vi "Profile Creation.vi"() -> ()   [LabVIEW 2018]
uses:
  Controls/Profile Create Cluster.ctl
panel:
  in  "Select Profile":path
  in  "Profile Creation":T1[](array[typedef])
  out "Headline":string
  in  "Save Button":bool
  # "Auto Cycle Profile Creation"
  # "Start RPM"
  # "End RPM"
  # "Ramp Time"
  # "Torque Value"
  # "Operation"
  # "Stable Time"
  # "Datalog"
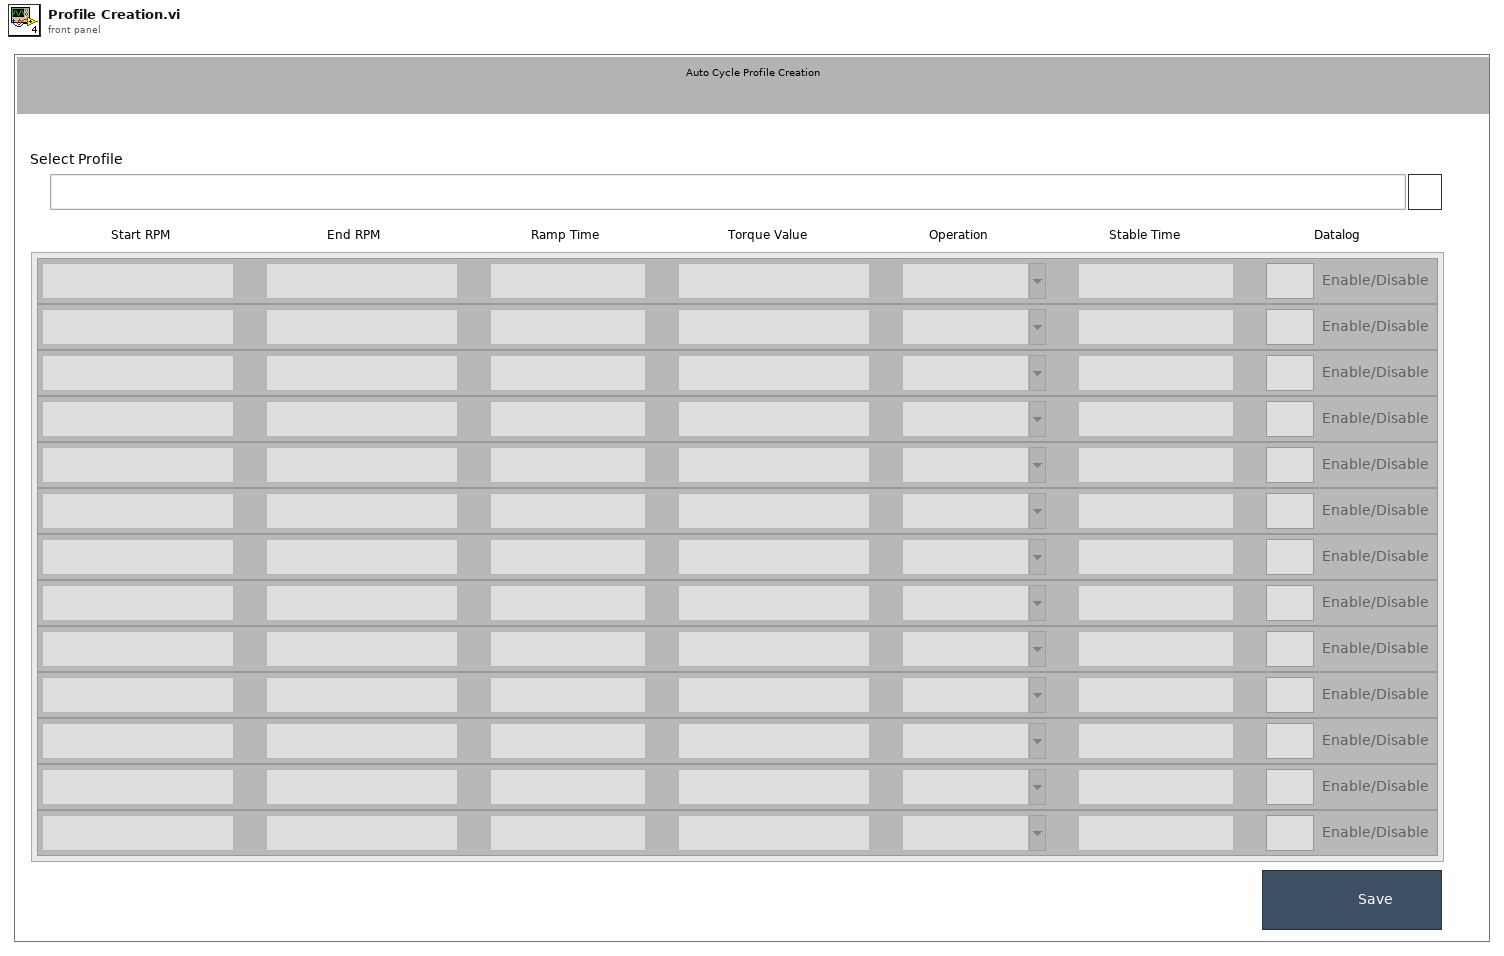
[diagram p1: front panel]
types:
  T1 = typedef "Profile Create Cluster.ctl" = cluster{"Start RPM":string, "End RPM":string, "Operation":string, "Torque Value":string, "Datalog":bool, "Ramp Time":string, "Stable Time":string}
  T2 = enum32{"Invalid", "Standard", "Closed", "Hidden", "Minimized", "Maximized"}
  T3 = enum32{"invalid app kind", "Development System", "Run Time System", "Student Edition", "Embedded LabVIEW", "Evaluation", "Custom"}
  T4 = cluster{"Core":cluster{"Current VI Reference":refnum<vi>, "Close Panel on Exit?":bool}, "Your Boolean data":bool, "Your string data":string, "Profile Creation":T1[], "File paths":cluster{"Base file path":path, "Model File path":path}, "Select Profile":path}
  T5 = cluster{"Base file path":path, "Model File path":path}
  T6 = cluster{"Current VI Reference":refnum<vi>, "Close Panel on Exit?":bool}
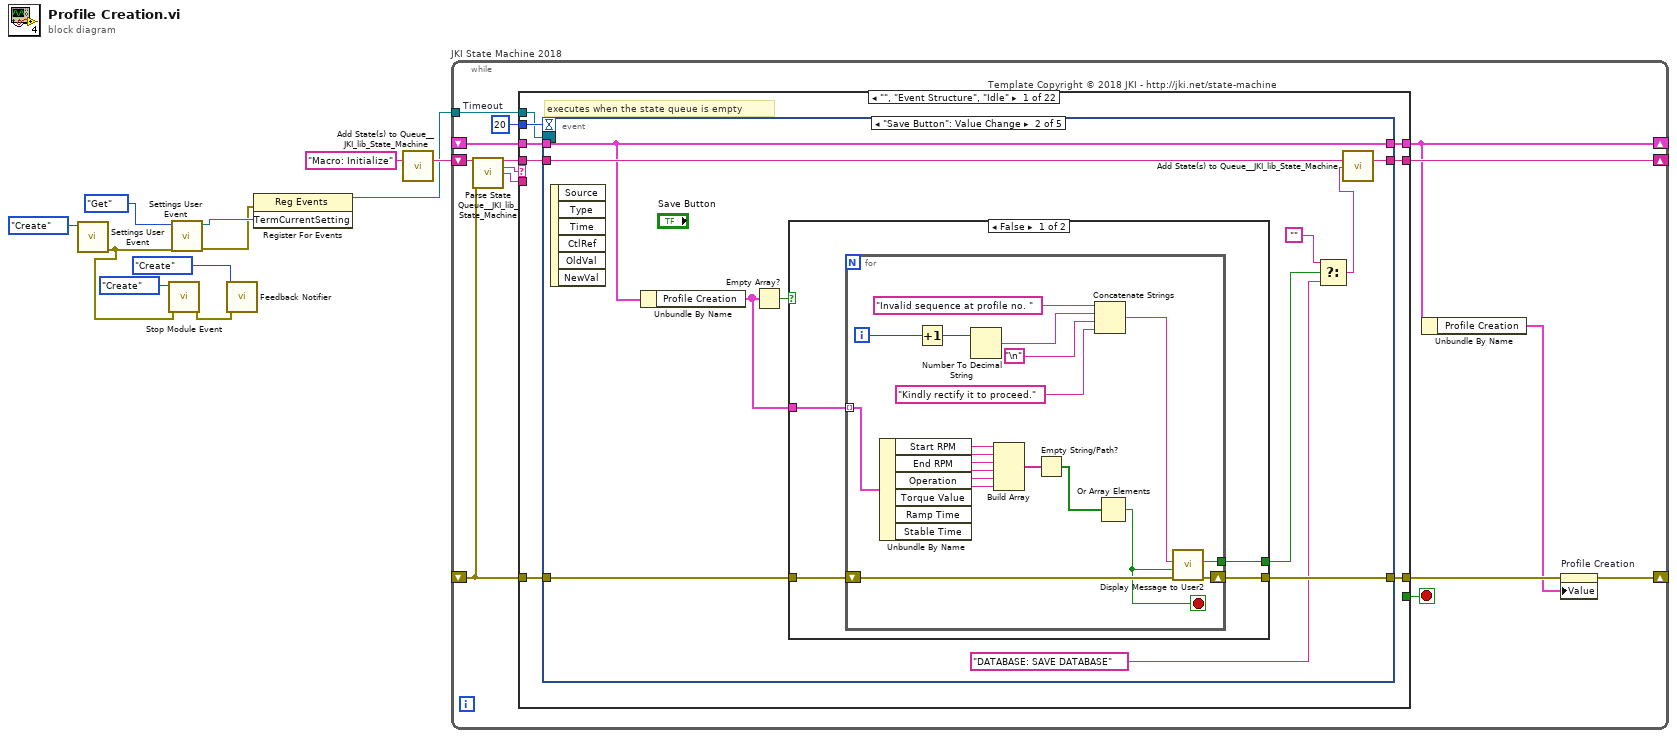
[diagram p0: block diagram]
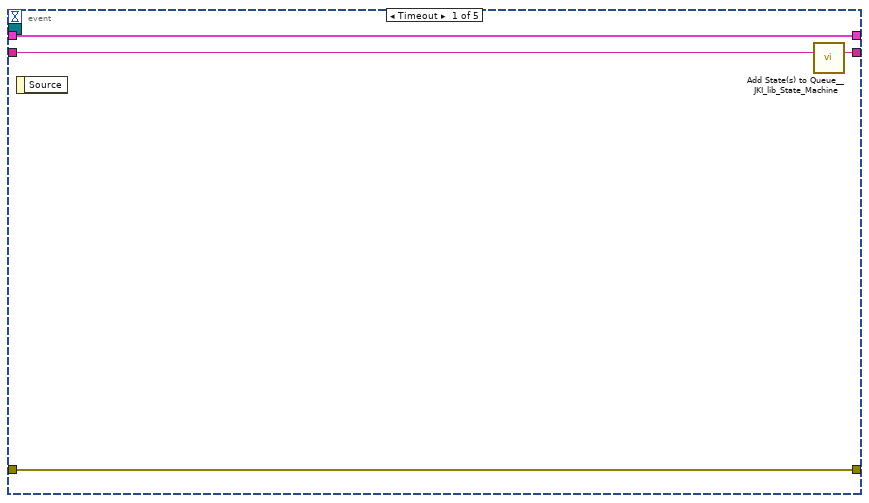
[diagram p2: hidden frame]
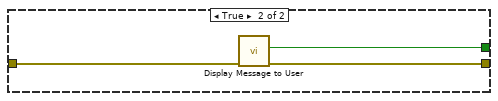
[diagram p3: hidden frame]
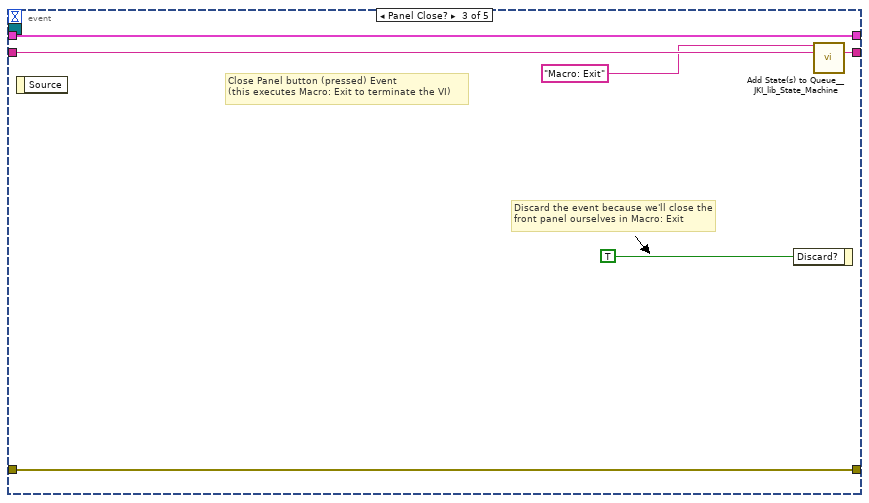
[diagram p4: hidden frame]
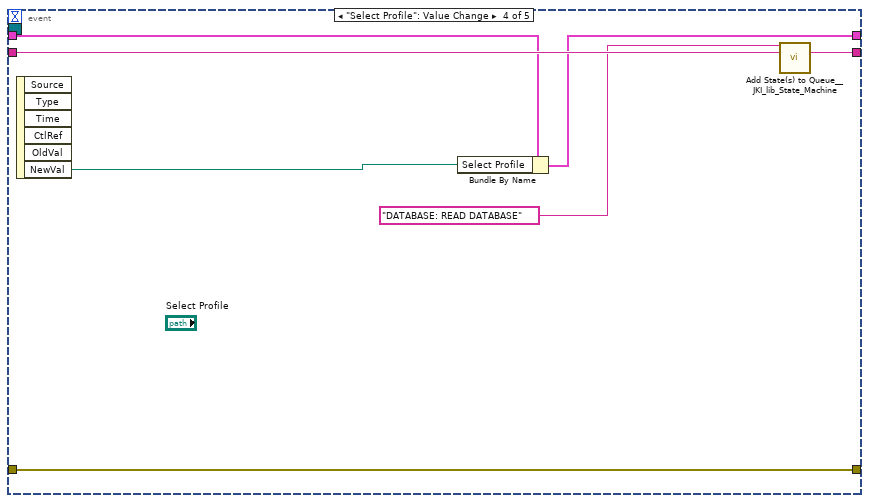
[diagram p5: hidden frame]
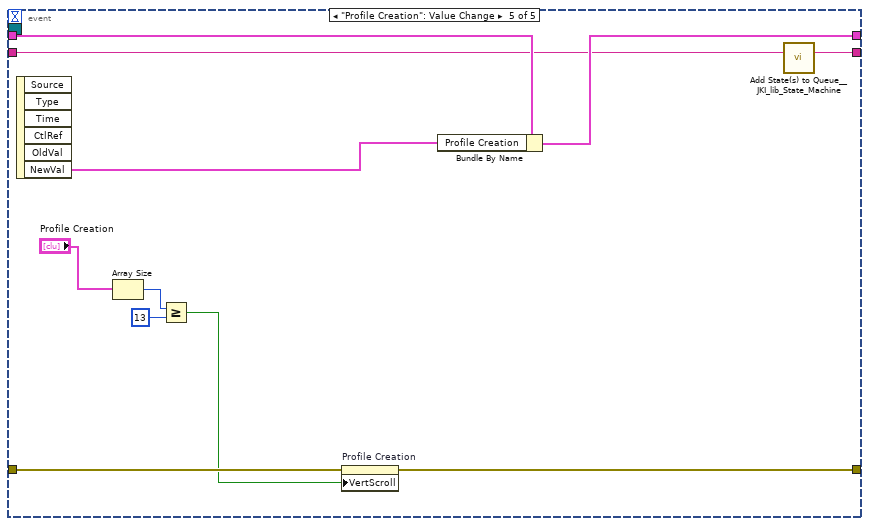
[diagram p6: hidden frame]
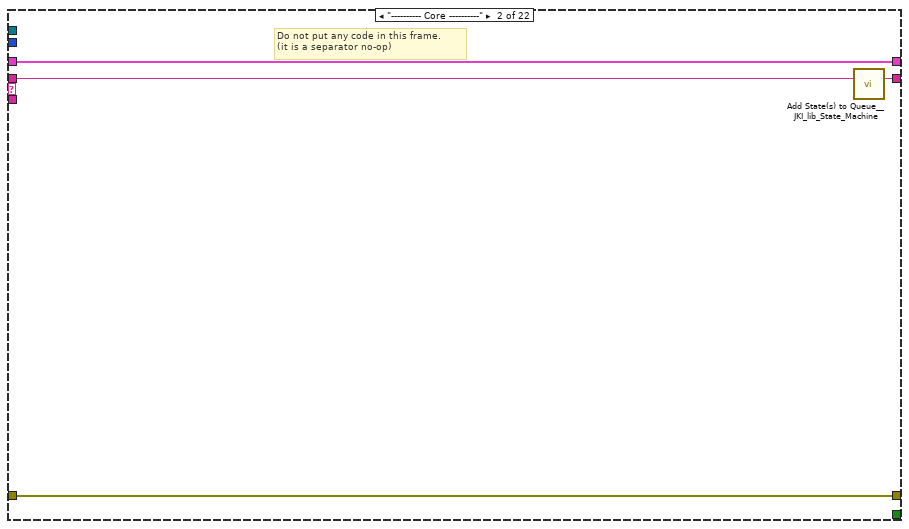
[diagram p7: hidden frame]
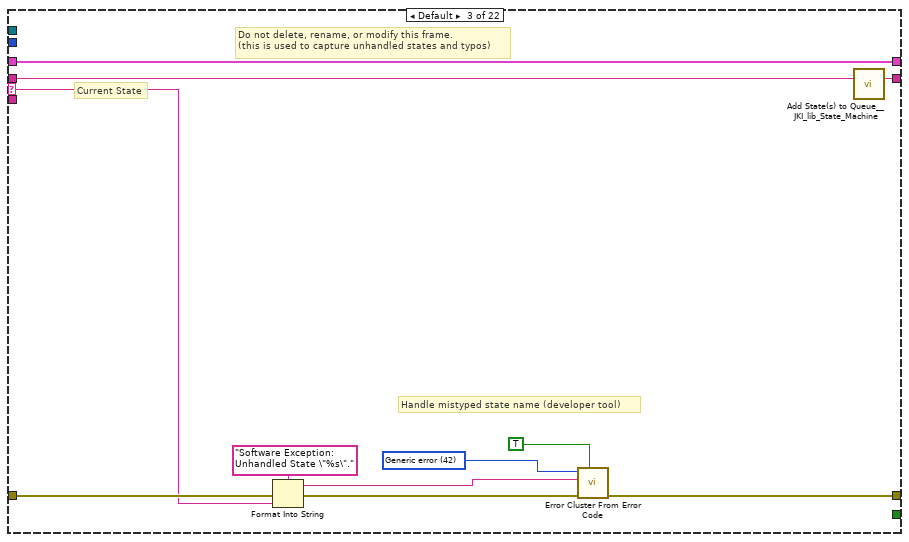
[diagram p8: hidden frame]
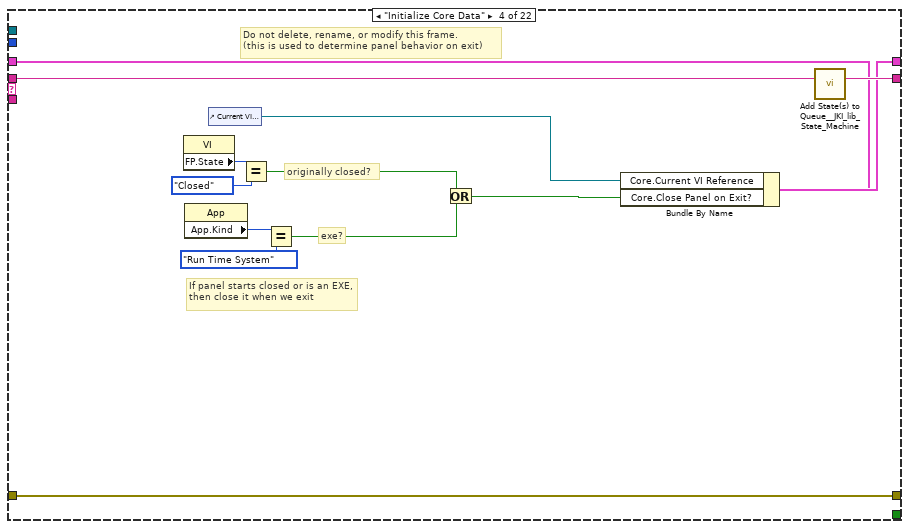
[diagram p9: hidden frame]
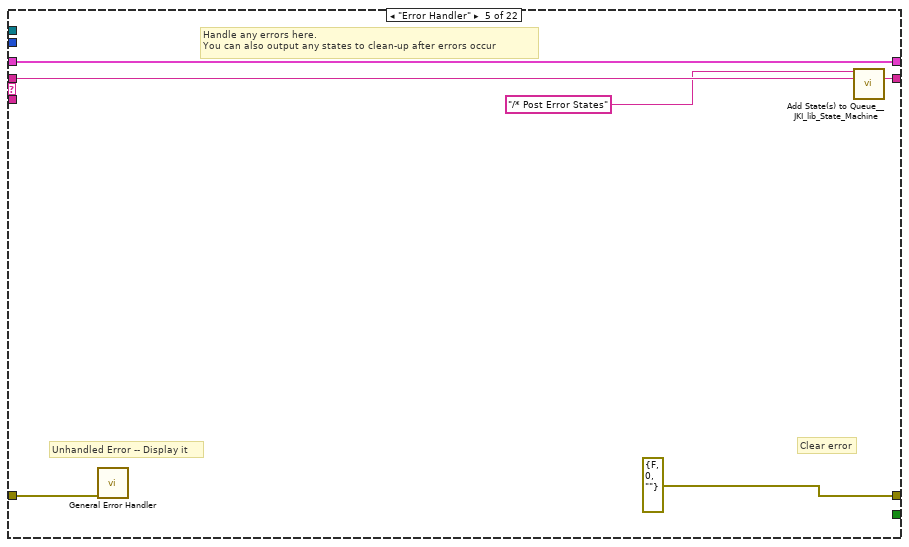
[diagram p10: hidden frame]
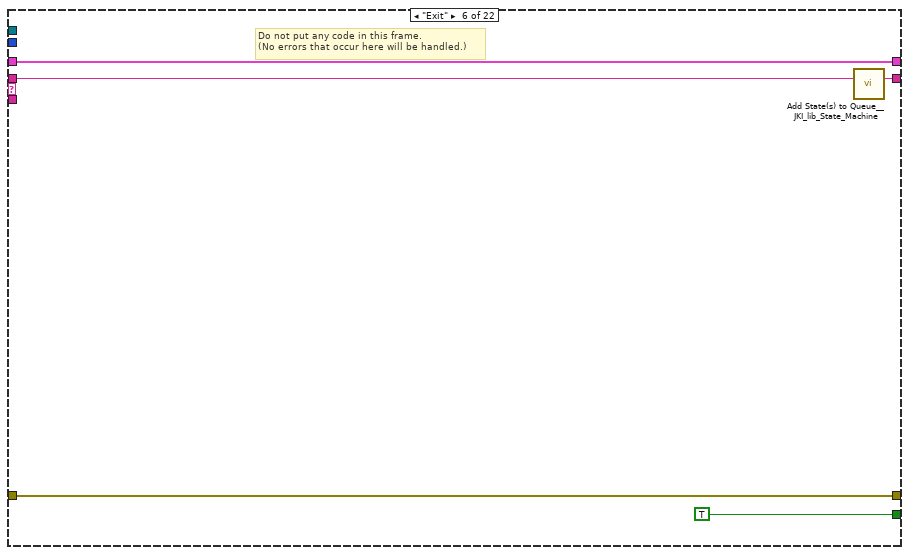
[diagram p11: hidden frame]
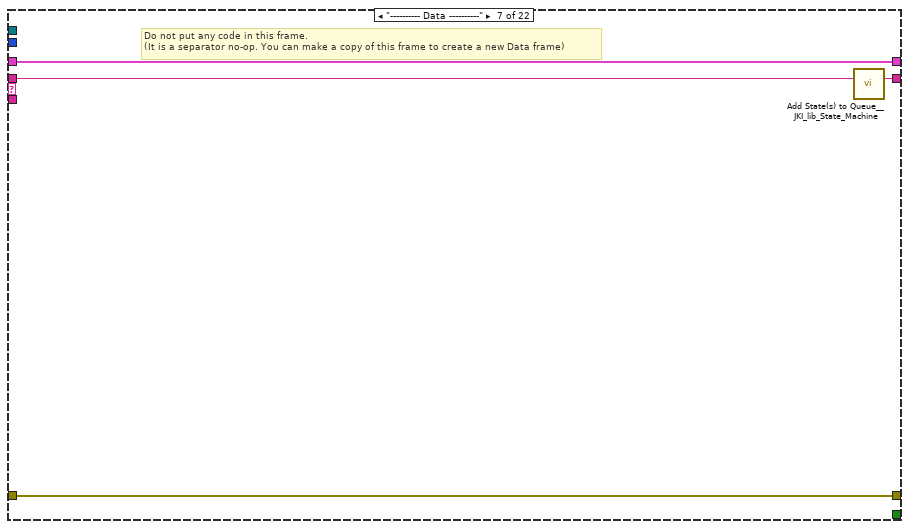
[diagram p12: hidden frame]
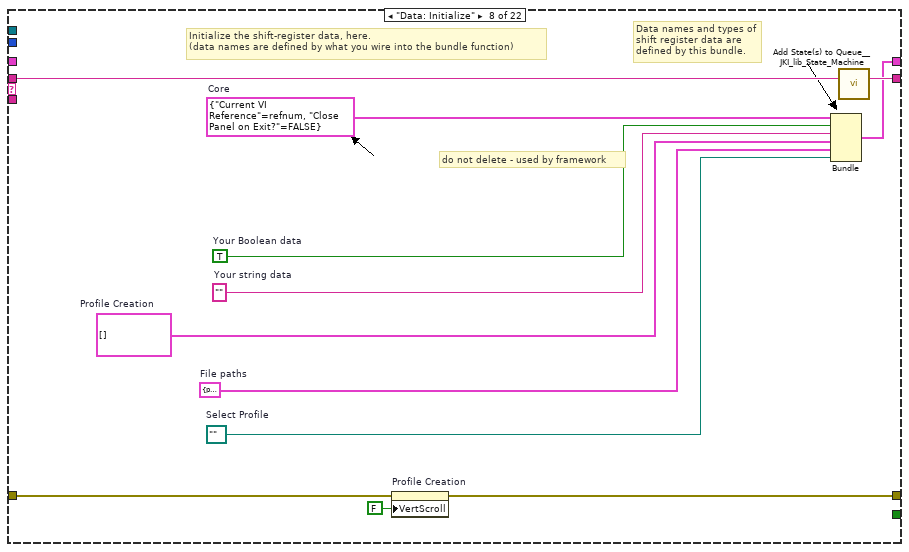
[diagram p13: hidden frame]
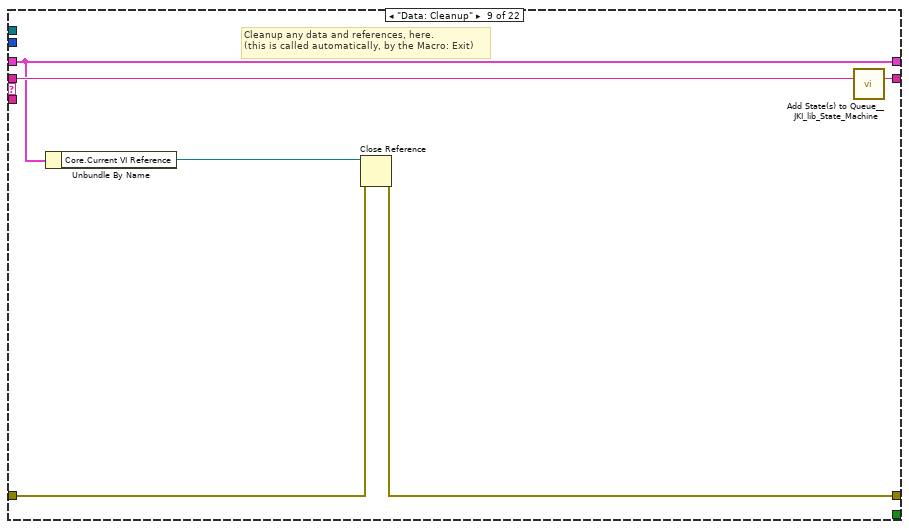
[diagram p14: hidden frame]
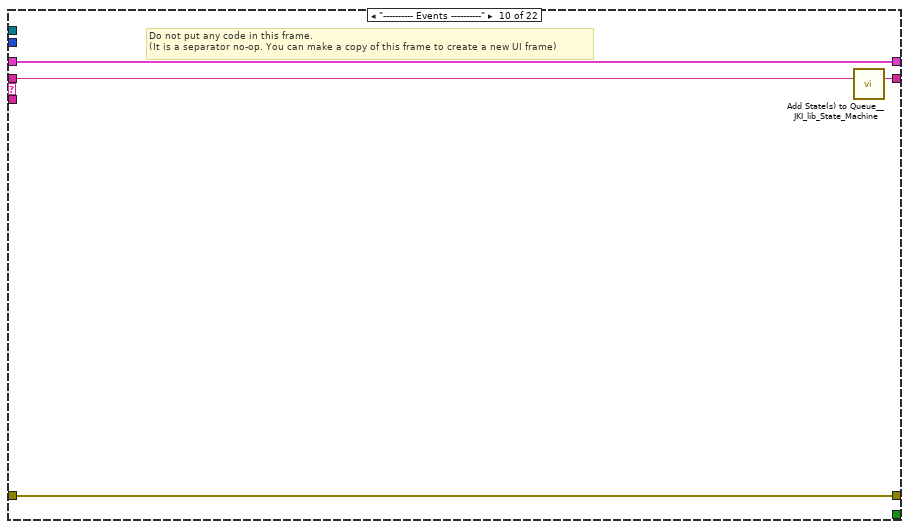
[diagram p15: hidden frame]
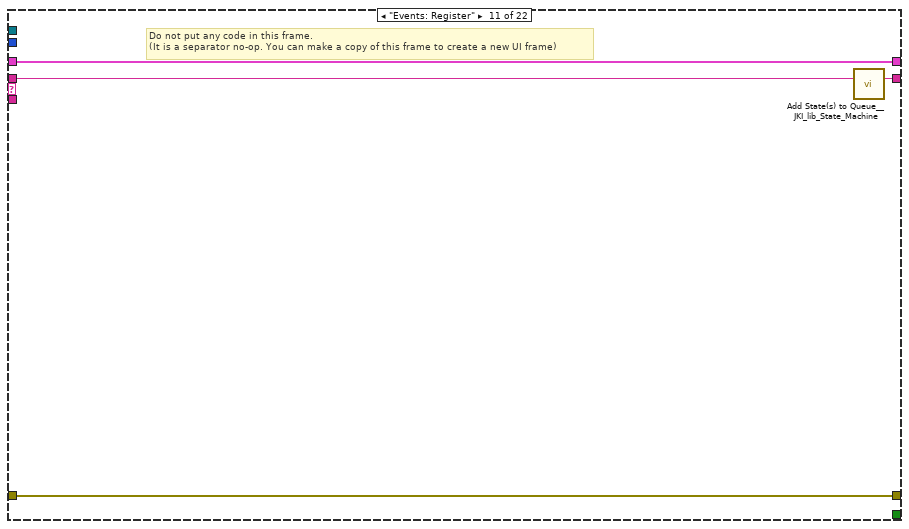
[diagram p16: hidden frame]
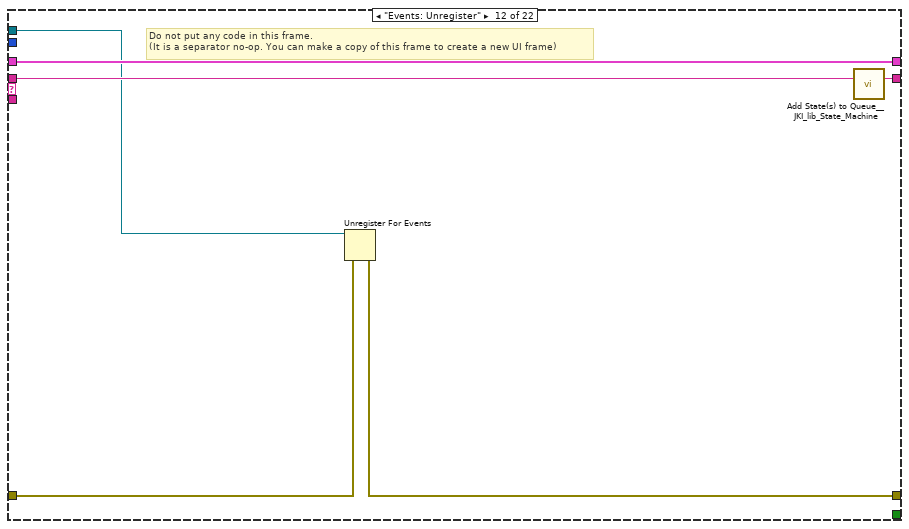
[diagram p17: hidden frame]
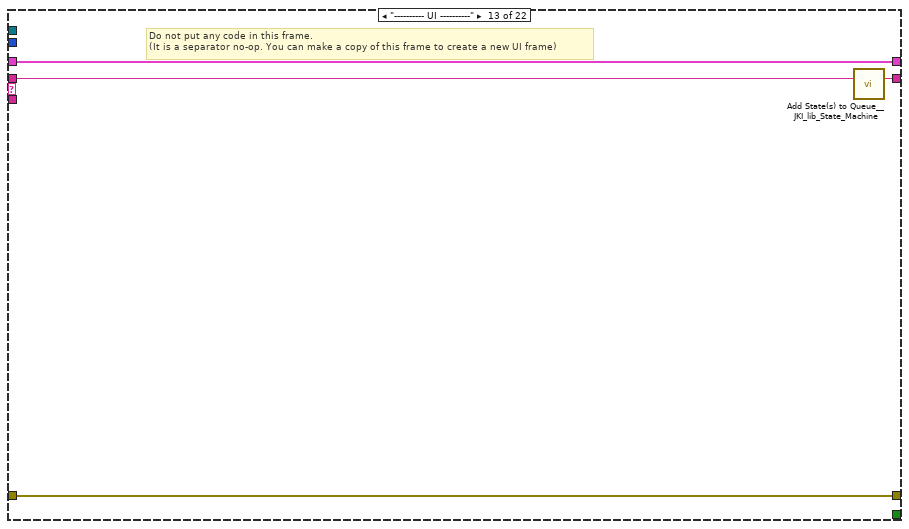
[diagram p18: hidden frame]
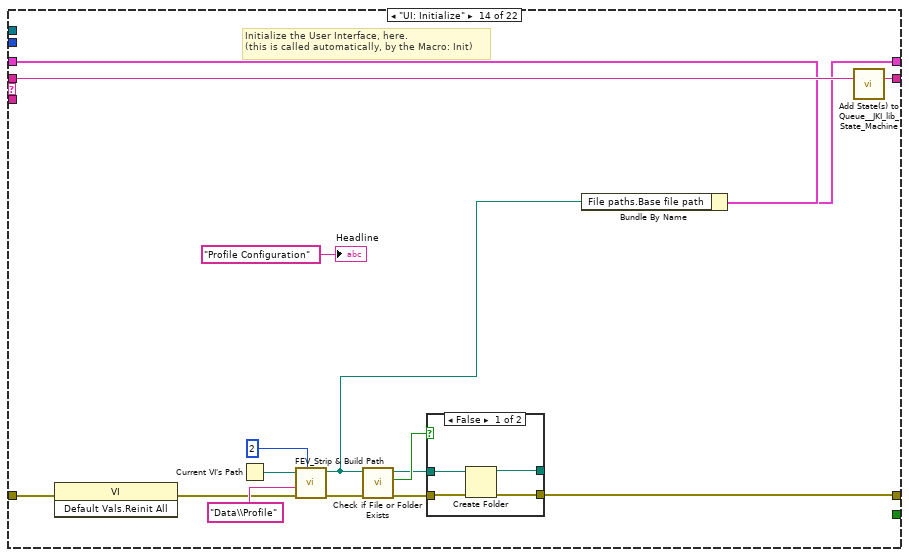
[diagram p19: hidden frame]
diagram:
  n1 = call "Settings User Event.vi"("Action"=enum16{"Create", "Get", "Destroy"}."Create") -> ("error out"=w4:errorcluster)  [unwired: 9 in, 1 out]
  n2 = call "Stop Module Event.vi"("error in (no error)"=w4, "Action"=enum16{"Create", "Get", "Destroy"}."Create") -> ("error out"=w3:errorcluster)  [unwired: 8 in, 1 out]
  n3 = call "Settings User Event.vi"("error in (no error)"=w4, "Action"=enum16{"Create", "Get", "Destroy"}."Get") -> ("error out"=w6:errorcluster, "TermCurrentSetting"=w7:refnum<user-event>)  [unwired: 8 in]
  n4 = call "Feedback Notifier.vi"("error in (no error)"=w3, "Action"=enum16{"Create", "Get", "Destroy"}."Create") -> ()  [unwired: 8 in, 2 out]
  n5 = register-events(error in=w6, w7) -> (reference out=w1:refnum<event-registration>)  [unwired: 1 in, 1 out]
  n6 = call <vilib>:"Add State(s) to Queue__JKI_lib_State_Machine.vi"("State(s) in (\"\")"="Macro: Initialize") -> ("States Out"=w11:string)  [unwired: 14 in]
  n7 = while "JKI State Machine 2018" {
    shift-right: [w13] -> _
    shift-left: _ -> [w19]
    shift-right: [w14] -> _
    shift-left: _ -> [w17]
    shift-right: [w21] -> _
    shift-left: w11 -> [w22]
    tunnel: w1 -> [w16]
    stop <- w20 stop-if-true
    w18 = 20  # Timeout
    # "Template Copyright © 2018 JKI - http://jki.net/state-machine"
    n8 = call <vilib>:"Parse State Queue__JKI_lib_State_Machine.vi"("State Queue"=w22, "Error In (no error)"=w17) -> ("Remaining States"=w24:string, "Current State"=w25:string, "Arguments"=w23:string)  [unwired: 11 in]
    n9 = case shown="\"\", \"Event Structure\", \"Idle\"" w25 {
      selector: w25 -> [_ _ w104 _ _ _ _ _ _ _ _ _ _ _ _ _ _ _ _ _ _ _]
      tunnel: w24 -> [w33 w103 w108 w127 w133 w138 w142 w154 w160 w164 w168 w174 w178 w194 w206 w217 w286 w291 w301 w305 w316 w340]
      tunnel: w23 -> [_ _ _ _ _ _ _ _ _ _ _ _ _ _ w201 w211 _ _ _ _ _ _]
      tunnel: w19 -> [w31 w100 w106 w120 w130 w136 w139 _ w155 w161 w166 w172 w175 w189 w204 w213 w283 w288 w298 w302 w314 w338]
      tunnel: [w30 w101 w110 w124 errorcluster {"status"=FALSE, "code"=0, "source"=""} ("error out") w135 w140 w143 w156 w162 w165 w169 w176 w179 w202 w214 w284 w289 w299 w303 w313 w331] -> w15
      tunnel: w17 -> [w29 w101 w109 w124 w129 w135 w140 w144 w157 w162 w165 w170 w176 w187 w203 w215 w284 w289 w299 w303 w310 w336]
      tunnel: [w32 w102 w107 w126 w132 w137 w141 w153 w159 w163 w167 w173 w177 w193 w205 w216 w285 w290 w300 w304 w315 w339] -> w21
      tunnel: [_ _ _ _ _ TRUE _ _ _ _ _ _ _ _ _ _ _ _ _ _ _ _] -> w20
      tunnel: [w28 w100 w106 w125 w130 w136 w139 w152 w155 w161 w166 w172 w175 w188 w204 w213 w283 w288 w298 w302 w314 w337] -> w13
      tunnel: w18 -> [w27 _ _ _ _ _ _ _ _ _ _ _ _ _ _ _ _ _ _ _ _ _]
      tunnel: w16 -> [w26 _ _ _ _ _ _ _ _ _ _ w171 _ _ _ _ _ _ _ _ _ _]
      frame "", "Event Structure", "Idle" {
        # "executes when the state queue is empty"
        n10 = event shown="[1] \"Save Button\": Value Change" {
          selector: w26 -> [_ _ _ _ _]
          dyn-events: _ -> [_ _ _ _ _]
          timeout: w27 -> [_ _ _ _ _]
          tunnel: w33 -> [w37 w47 w81 w86 w96]
          tunnel: [w36 w48 w80 w87 w97] -> w32
          tunnel: w31 -> [w34 w46 w78 w85 w99]
          tunnel: [w35 w43 w79 w88 w91] -> w30
          tunnel: w29 -> [w35 w45 w79 w88 w92]
          tunnel: [w34 w46 w78 w84 w98] -> w28
          event Timeout {
            n11 = event-data() -> ()  [unwired: 1 in, 1 out]
            n12 = call <vilib>:"Add State(s) to Queue__JKI_lib_State_Machine.vi"("State(s) in (\"\")"=w37) -> ("States Out"=w36:string)  [unwired: 14 in]
          }
          event "Save Button": Value Change {
            n13 = event-data() -> ()  [unwired: 1 in, 6 out]
            n14 = Unbundle By Name(w46) -> ("Profile Creation"=w42:T1[])
            n15 = Empty Array?(array=w42) -> (empty?=w44:bool)
            n16 = case shown="False" w44 {
              tunnel: w45 -> [w51 w75]
              tunnel: [w50 w74] -> w43
              tunnel: w42 -> [w52 _]
              tunnel: [w49 w73] -> w41
              frame False {
                n17 = for {
                  tunnel: w52 -> [w72] mode=indexing
                  shift-right: [w63] -> w50
                  shift-left: w51 -> [w64]
                  tunnel: [w53] -> w49
                  i -> [w60]
                  stop <- w61 stop-if-true
                  n18 = Unbundle By Name(w72) -> ("Start RPM"=w71:string, "End RPM"=w70:string, "Operation"=w69:string, "Torque Value"=w68:string, "Ramp Time"=w67:string, "Stable Time"=w66:string)
                  n19 = Increment(x=w60) -> (x+1=w59:i32)
                  n20 = Number To Decimal String(number=w59) -> (decimal integer string=w58:string)  [unwired: 1 in]
                  n21 = Build Array(w71, w70, w69, w68, w67, w66) -> (w65:string[])
                  n22 = Empty String/Path?(string/path=w65) -> (empty?=w62:bool[])
                  n23 = Concatenate Strings("Invalid sequence at profile no. " ("string"), w58, "\n", "Kindly rectify it to proceed." ("string")) -> (w55:string)
                  n24 = Or Array Elements(Boolean array=w62) -> (logical OR=w61:bool)
                  n25 = call "Display Message to User2"("error in (no error)"=w64, "Enable"=w61, "Message"=w55) -> ("error out"=w63:errorcluster, "OK"=w53:bool)  [unwired: 7 in]
                }
              }
              frame True {
                n26 = call "Display Message to User"("error in (no error)"=w75) -> ("error out"=w74:errorcluster, "OK"=w73:bool)  [unwired: 9 in]
              }
            }
            n27 = Select(t="", s=w41, f="DATABASE: SAVE DATABASE") -> (s? t:f=w38:string)
            n28 = call <vilib>:"Add State(s) to Queue__JKI_lib_State_Machine.vi"("State(s) in (\"\")"=w47, "State(s) at Back (\"\")"=w38) -> ("States Out"=w48:string)  [unwired: 13 in]
          }
          event Panel Close? {
            # "Discard the event because we'll close the front panel ourselves in Macro: Exit"
            # "Close Panel button (pressed) Event\n(this executes Macro: Exit to terminate the VI)"
            n29 = event-data() -> ()  [unwired: 1 in, 1 out]
            n30 = event-data("Discard?"=TRUE) -> ()  [unwired: 1 in, 1 out]
            n31 = call <vilib>:"Add State(s) to Queue__JKI_lib_State_Machine.vi"("State(s) in Front (\"\")"="Macro: Exit", "State(s) in (\"\")"=w81) -> ("States Out"=w80:string)  [unwired: 13 in]
          }
          event "Select Profile": Value Change {
            n32 = event-data() -> ("NewVal"=w83:path)  [unwired: 1 in, 5 out]
            n33 = Bundle By Name(cluster=w85, "Select Profile"=w83) -> (w84:T4)
            n34 = call <vilib>:"Add State(s) to Queue__JKI_lib_State_Machine.vi"("State(s) in Front (\"\")"="DATABASE: READ DATABASE" ("State(s) in Front (\"\")"), "State(s) in (\"\")"=w86) -> ("States Out"=w87:string)  [unwired: 13 in]
          }
          event "Profile Creation": Value Change {
            n35 = event-data() -> ("NewVal"=w89:T1[])  [unwired: 1 in, 5 out]
            n36 = Array Size(array="Profile Creation") -> (size(s)=w94:i32)
            n37 = Greater Or Equal?(x=w94, y=13) -> (x >= y?=w90:bool)
            n38 = property on="Profile Creation" class="Arr (strict)"(error in=w92, "VertScroll"=w90) -> (error out=w91:errorcluster)  [unwired: 1 in, 1 out]
            n39 = Bundle By Name(cluster=w99, "Profile Creation"=w89) -> (w98:T4)
            n40 = call <vilib>:"Add State(s) to Queue__JKI_lib_State_Machine.vi"("State(s) in (\"\")"=w96) -> ("States Out"=w97:string)  [unwired: 14 in]
          }
        }
      }
      frame "---------- Core ----------" {
        # "Do not put any code in this frame.\n(it is a separator no-op)"
        n41 = call <vilib>:"Add State(s) to Queue__JKI_lib_State_Machine.vi"("State(s) in (\"\")"=w103) -> ("States Out"=w102:string)  [unwired: 14 in]
      }
      frame Default {
        w113 = 42 items=["No error", "Argument error", "Memory is full", "Out of zone", "End of file", "File already open", "Generic file I/O error", "File not found", "File permission error", "Disk is full", "Duplicate path", "Too many files open", "System feature not enabled", "Resource file not found", "Cannot add resource", "Resource not found", "Image not found", "Image memory error", "Pen does not exist", "Config type invalid", "Config token not found", "Config parse error", "Config memory error", "Bad external code format", "Bad external code offset", "External code not present", "Null window", "Destroy window error", "Null menu", "Print aborted", "Bad print record", "Print driver error", "Windows error during printing", "Memory error during printing", "Print dialog error", "Generic print error", "Invalid device refnum", "Device not found", "Device parameter error", "Device unit error", "Cannot open device", "Device call aborted", "Generic error", "Cancelled by user", "Object ID too low", "Object ID too high", "Object not in heap", "Unknown heap", "Unknown object (invalid DefProc)", "Unknown object (DefProc not in table)", "Message out of range", "Invalid (null) method", "Unknown message", "Manager call not supported", "Bad address", "Network operation in progress", "Network operation timed out", "Connection is busy", "Network attribute not supported", "Network error", "Address in use", "System out of memory", "Connection aborted", "Connection refused", "Not connected", "Already connected", "Connection closed", "Initialization error (interapplication manager)", "Bad occurrence", "Wait on unbound occurrence handler", "Occurrence queue overflow", "Datalog type conflict", "Unused", "Unrecognized type (interapplication manager)", "Memory corrupt", "Failed to make temporary DLL", "Old CIN version", "Drag socket not found", "Failed to load drop-object", "Failed to register OLE object", "Failed to release OLE object", "Format specifier type mismatch", "Unknown format specifier", "Too few format specifiers", "Too many format specifiers", "Scan failed", "Newer CIN version", "Error converting to variant", "Runtime menu error", "Password tampered", "Variant attribute not found", "Incompatible variant data type", "Event data is not available", "Event Store is not present", "Occurrence is not found", "Event Queue is not created", "Event info is not available", "Refnum passed is NULL", "Error retrieving Class GUID", "Error retrieving CoClass GUID", "Error retrieving TypeLib GUID.", "Bad built application magic bytes.", "Specific driver is different from the specific driver associated with the Logical Name.", "There is no session opened to the class driver.", "Max Error", "MAX - Error with config objects", "MAX - Error loading configuration", "MAX - Group not supported"]
        # "Current State"
        # "Do not delete, rename, or modify this frame.\n(this is used to capture unhandled states and typos)"
        # "Handle mistyped state name (developer tool)"
        n42 = Format Into String(format string="Software Exception: Unhandled State \"%s\"." ("message"), error in=w109, w104) -> (resulting string=w112:string, error out=w111:errorcluster)  [unwired: 1 in]
        n43 = call <vilib>:"Error Cluster From Error Code.vi"("show call chain? (False)"=TRUE, "error in (no error)"=w111, "error message (\"\")"=w112, "error code (0)"=w113) -> ("error out"=w110:errorcluster)  [unwired: 5 in]
        n44 = call <vilib>:"Add State(s) to Queue__JKI_lib_State_Machine.vi"("State(s) in (\"\")"=w108) -> ("States Out"=w107:string)  [unwired: 14 in]
      }
      frame "Initialize Core Data" {
        # "Do not delete, rename, or modify this frame.\n(this is used to determine panel behavior on exit)"
        # "originally closed?"
        # "exe?"
        # "If panel starts closed or is an EXE, then close it when we exit"
        n45 = property class="VI"() -> ("FP.State"=w117:T2)  [unwired: 2 in, 2 out]
        n46 = property class="App"() -> ("App.Kind"=w123:T3)  [unwired: 2 in, 2 out]
        n47 = control-ref of="Current VI Reference"() -> (w118:refnum<vi>)
        n48 = Equal?(x=w117, y=T2."Closed" ("Front Panel Window:State")) -> (x = y?=w115:bool)
        n49 = Equal?(x=w123, y=T3."Run Time System" ("Application:Kind")) -> (x = y?=w121:bool)
        n50 = Or(x=w115, y=w121) -> (x .or. y?=w119:bool)
        n51 = Bundle By Name(cluster=w120, "Core.Current VI Reference"=w118, "Core.Close Panel on Exit?"=w119) -> (w125:T4)
        n52 = call <vilib>:"Add State(s) to Queue__JKI_lib_State_Machine.vi"("State(s) in (\"\")"=w127) -> ("States Out"=w126:string)  [unwired: 14 in]
      }
      frame "Error Handler" {
        # "Unhandled Error -- Display it"
        # "Handle any errors here.\nYou can also output any states to clean-up after errors occur"
        # "Clear error"
        n53 = call <vilib>:"General Error Handler.vi"("error in (no error)"=w129) -> ()  [unwired: 10 in, 5 out]
        n54 = call <vilib>:"Add State(s) to Queue__JKI_lib_State_Machine.vi"("State(s) in Front (\"\")"="/* Post Error States", "State(s) in (\"\")"=w133) -> ("States Out"=w132:string)  [unwired: 13 in]
      }
      frame "Exit" {
        # "Do not put any code in this frame.\n(No errors that occur here will be handled.)"
        n55 = call <vilib>:"Add State(s) to Queue__JKI_lib_State_Machine.vi"("State(s) in (\"\")"=w138) -> ("States Out"=w137:string)  [unwired: 14 in]
      }
      frame "---------- Data ----------" {
        # "Do not put any code in this frame.\n(It is a separator no-op. You can make a copy of this frame to create a new Data frame)"
        n56 = call <vilib>:"Add State(s) to Queue__JKI_lib_State_Machine.vi"("State(s) in (\"\")"=w142) -> ("States Out"=w141:string)  [unwired: 14 in]
      }
      frame "Data: Initialize" {
        w146 = T1[] []  # Profile Creation
        w147 = path ""  # Select Profile
        w148 = T5 {"Base file path"=path "", "Model File path"=path ""}  # File paths
        w149 = T6 {"Current VI Reference"=refnum, "Close Panel on Exit?"=FALSE}  # Core
        w151 = TRUE  # Your Boolean data
        w150 = ""  # Your string data
        # "do not delete - used by framework"
        # "Data names and types of shift register data are defined by this bundle."
        # "Initialize the shift-register data, here.\n(data names are defined by what you wire into the bundle function)"
        n57 = property on="Profile Creation" class="Arr (strict)"(error in=w144, "VertScroll"=FALSE ("Vertical Scrollbar Visible")) -> (error out=w143:errorcluster)  [unwired: 1 in, 1 out]
        n58 = Bundle("Core"=w149, "Your Boolean data"=w151, "Your string data"=w150, "Profile Creation"=w146, "File paths"=w148, "Select Profile"=w147) -> (w152:T4)  [unwired: 1 in]
        n59 = call <vilib>:"Add State(s) to Queue__JKI_lib_State_Machine.vi"("State(s) in (\"\")"=w154) -> ("States Out"=w153:string)  [unwired: 14 in]
      }
      frame "Data: Cleanup" {
        # "Cleanup any data and references, here.\n(this is called automatically, by the Macro: Exit)"
        n60 = Unbundle By Name(w155) -> ("Core.Current VI Reference"=w158:refnum<vi>)
        n61 = Close Reference(reference=w158, error in (no error)=w157) -> (error out=w156:errorcluster)
        n62 = call <vilib>:"Add State(s) to Queue__JKI_lib_State_Machine.vi"("State(s) in (\"\")"=w160) -> ("States Out"=w159:string)  [unwired: 14 in]
      }
      frame "---------- Events ----------" {
        # "Do not put any code in this frame.\n(It is a separator no-op. You can make a copy of this frame to create a new UI frame)"
        n63 = call <vilib>:"Add State(s) to Queue__JKI_lib_State_Machine.vi"("State(s) in (\"\")"=w164) -> ("States Out"=w163:string)  [unwired: 14 in]
      }
      frame "Events: Register" {
        # "Do not put any code in this frame.\n(It is a separator no-op. You can make a copy of this frame to create a new UI frame)"
        n64 = call <vilib>:"Add State(s) to Queue__JKI_lib_State_Machine.vi"("State(s) in (\"\")"=w168) -> ("States Out"=w167:string)  [unwired: 14 in]
      }
      frame "Events: Unregister" {
        # "Do not put any code in this frame.\n(It is a separator no-op. You can make a copy of this frame to create a new UI frame)"
        n65 = Unregister For Events(event registration refnum=w171, error in=w170) -> (error out=w169:errorcluster)
        n66 = call <vilib>:"Add State(s) to Queue__JKI_lib_State_Machine.vi"("State(s) in (\"\")"=w174) -> ("States Out"=w173:string)  [unwired: 14 in]
      }
      frame "---------- UI ----------" {
        # "Do not put any code in this frame.\n(It is a separator no-op. You can make a copy of this frame to create a new UI frame)"
        n67 = call <vilib>:"Add State(s) to Queue__JKI_lib_State_Machine.vi"("State(s) in (\"\")"=w178) -> ("States Out"=w177:string)  [unwired: 14 in]
      }
      frame "UI: Initialize" {
        # "Initialize the User Interface, here.\n(this is called automatically, by the Macro: Init)"
        n68 = invoke class="VI" method="Default Vals.Reinit All"(error in=w187) -> (error out=w186:errorcluster)  [unwired: 2 in, 2 out]
        n69 = Current VI's Path() -> (path=w191:path)
        n70 = call "FEV_Strip & Build Path.vi"("Strip Levels"=2, "error in (no error)"=w186, "Build Path"="Data\\Profile", "Path In"=w191) -> ("error out"=w184:errorcluster, "New Path Out"=w183:path)  [unwired: 5 in, 1 out]
        n71 = call <vilib>:"Check if File or Folder Exists.vi"("error in (no error)"=w184, "path"=w183) -> ("error out"=w182:errorcluster, "file or folder exists?"=w181:bool, "dup path"=w180:path)  [unwired: 7 in]
        n72 = case shown="False" w181 {
          tunnel: w182 -> [w197 w199]
          tunnel: w180 -> [w198 w200]
          tunnel: [w196 w199] -> w179
          tunnel: [w195 w200] -> _
          frame False {
            n73 = Create Folder(path (use dialog)=w198, error in=w197) -> (created path=w195:path, error out=w196:errorcluster)  [unwired: 1 in, 1 out]
          }
          frame True {
          }
        }
        n74 = Bundle By Name(cluster=w189, "File paths.Base file path"=w183) -> (w188:T4)
        n75 = call <vilib>:"Add State(s) to Queue__JKI_lib_State_Machine.vi"("State(s) in (\"\")"=w194) -> ("States Out"=w193:string)  [unwired: 14 in]
        "Headline" <- "Profile Configuration" ("Headline")
      }
      frame "UI: Cursor Set" {
        # "Argument"
        # "Set and Unset Cursor Busy.\n(Usage: \"UI: Cursor Set >> Busy|Idle\")"
        n76 = case shown="\"Idle\", Default" w201 {
          tunnel: w203 -> [w208 w210]
          tunnel: [w207 w209] -> w202
          frame "Idle", Default {
            n77 = call <vilib>:"Unset Busy.vi"("error in (no error)"=w208) -> ("error out"=w207:errorcluster)  [unwired: 10 in]
          }
          frame "Busy" {
            n78 = call <vilib>:"Set Busy.vi"("error in (no error)"=w210) -> ("error out"=w209:errorcluster)  [unwired: 9 in, 1 out]
          }
        }
        n79 = call <vilib>:"Add State(s) to Queue__JKI_lib_State_Machine.vi"("State(s) in (\"\")"=w206) -> ("States Out"=w205:string)  [unwired: 14 in]
      }
      frame "UI: Front Panel State" {
        # "Argument"
        # "Set Front Panel Open or Closed\n(Usage: \"UI: Front Panel State >> Open|Close\")"
        n80 = Unbundle By Name(w213) -> ("Core.Current VI Reference"=w212:refnum<vi>)
        n81 = case shown="\"Open\", \"Standard\", Default" w211 {
          tunnel: w215 -> [w223 w238 w249 w262 w275]
          tunnel: [w225 w239 w251 w264 w277] -> w214
          tunnel: w212 -> [w224 w236 w250 w263 w276]
          frame "Open", "Standard", Default {
            w218 = T2."Standard" ("State")
            n82 = property class="VI"(reference=w224, error in=w223) -> (reference out=w221:refnum<vi>, error out=w222:errorcluster, "FP.State"=w220:T2)
            n83 = Not Equal?(x=w220, y=w218) -> (x != y?=w219:bool)
            n84 = case shown="True" w219 {
              tunnel: [w229 w231] -> w225
              tunnel: w222 -> [w228 w231]
              tunnel: w221 -> [w227 _]
              tunnel: w218 -> [w226 _]
              frame True {
                n85 = invoke class="VI" method="FP.Open"(reference=w227, error in=w228, "Activate"=TRUE, "State"=w226) -> (error out=w229:errorcluster)  [unwired: 1 in, 4 out]
              }
              frame False {
              }
            }
          }
          frame "Close", "Closed" {
            n86 = property class="VI"(reference=w236, error in=w238) -> (reference out=w235:refnum<vi>, error out=w237:errorcluster, "FP.State"=w233:T2)
            n87 = Not Equal?(x=w233, y=T2."Closed" ("Front Panel Window:State")) -> (x != y?=w232:bool)
            n88 = case shown="True" w232 {
              tunnel: [w240 w243] -> w239
              tunnel: w237 -> [w240 w242]
              tunnel: w235 -> [_ w241]
              frame False {
              }
              frame True {
                n89 = invoke class="VI" method="FP.Close"(reference=w241, error in=w242) -> (error out=w243:errorcluster)  [unwired: 1 in, 2 out]
              }
            }
          }
          frame "Hidden", "Hide" {
            w244 = T2."Hidden" ("State")
            n90 = property class="VI"(reference=w250, error in=w249) -> (reference out=w247:refnum<vi>, error out=w248:errorcluster, "FP.State"=w246:T2)
            n91 = Not Equal?(x=w246, y=w244) -> (x != y?=w245:bool)
            n92 = case shown="True" w245 {
              tunnel: [w255 w256] -> w251
              tunnel: w248 -> [w254 w256]
              tunnel: w247 -> [w253 _]
              tunnel: w244 -> [w252 _]
              frame True {
                n93 = invoke class="VI" method="FP.Open"(reference=w253, error in=w254, "State"=w252) -> (error out=w255:errorcluster)  [unwired: 2 in, 4 out]
              }
              frame False {
              }
            }
          }
          frame "Minimize", "Minimized" {
            w257 = T2."Minimized" ("State")
            n94 = property class="VI"(reference=w263, error in=w262) -> (reference out=w260:refnum<vi>, error out=w261:errorcluster, "FP.State"=w259:T2)
            n95 = Not Equal?(x=w259, y=w257) -> (x != y?=w258:bool)
            n96 = case shown="True" w258 {
              tunnel: [w268 w269] -> w264
              tunnel: w261 -> [w267 w269]
              tunnel: w260 -> [w266 _]
              tunnel: w257 -> [w265 _]
              frame True {
                n97 = invoke class="VI" method="FP.Open"(reference=w266, error in=w267, "State"=w265) -> (error out=w268:errorcluster)  [unwired: 2 in, 4 out]
              }
              frame False {
              }
            }
          }
          frame "Maximize", "Maximized" {
            w270 = T2."Maximized" ("State")
            n98 = property class="VI"(reference=w276, error in=w275) -> (reference out=w273:refnum<vi>, error out=w274:errorcluster, "FP.State"=w272:T2)
            n99 = Not Equal?(x=w272, y=w270) -> (x != y?=w271:bool)
            n100 = case shown="True" w271 {
              tunnel: [w281 w282] -> w277
              tunnel: w274 -> [w280 w282]
              tunnel: w273 -> [w279 _]
              tunnel: w270 -> [w278 _]
              frame True {
                n101 = invoke class="VI" method="FP.Open"(reference=w279, error in=w280, "State"=w278) -> (error out=w281:errorcluster)  [unwired: 2 in, 4 out]
              }
              frame False {
              }
            }
          }
        }
        n102 = call <vilib>:"Add State(s) to Queue__JKI_lib_State_Machine.vi"("State(s) in (\"\")"=w217) -> ("States Out"=w216:string)  [unwired: 14 in]
      }
      frame "---------- Macro ----------" {
        # "Do not put any code in this frame.\n(It is a separator no-op. You can make a copy of this frame to create a new Macro frame)"
        n103 = call <vilib>:"Add State(s) to Queue__JKI_lib_State_Machine.vi"("State(s) in (\"\")"=w286) -> ("States Out"=w285:string)  [unwired: 14 in]
      }
      frame "Macro: Initialize" {
        # "Initialization Macro\n(This is called once, when the VI starts)"
        n104 = call <vilib>:"Add State(s) to Queue__JKI_lib_State_Machine.vi"("State(s) in Front (\"\")"="Data: Initialize\nInitialize Core Data\nEvents: Register\nUI: Initialize\nUI: Front Panel State >> Open", "State(s) in (\"\")"=w291) -> ("States Out"=w290:string)  [unwired: 13 in]
      }
      frame "Macro: Exit" {
        # "Exit Macro\n(This is called once, when the VI exits)"
        n105 = Unbundle By Name(w298) -> ("Core.Close Panel on Exit?"=w297:bool)
        n106 = Select(t="UI: Front Panel State >> Close", s=w297, f="") -> (s? t:f=w294:string)
        n107 = call <vilib>:"Add State(s) to Queue__JKI_lib_State_Machine.vi"("State(s) in (\"\")"=w294, "State(s) at Back (\"\")"="Data: Cleanup\nEvents: Unregister\nExit") -> ("States Out"=w292:string)  [unwired: 13 in]
        n108 = call <vilib>:"Add State(s) to Queue__JKI_lib_State_Machine.vi"("State(s) in Front (\"\")"=w292, "State(s) in (\"\")"=w301) -> ("States Out"=w300:string)  [unwired: 13 in]
      }
      frame "---------- DATABSE ----------" {
        # "Template Separator\n(You can make a copy of, or modify, this frame)"
        n109 = call <vilib>:"Add State(s) to Queue__JKI_lib_State_Machine.vi"("State(s) in (\"\")"=w305) -> ("States Out"=w304:string)  [unwired: 14 in]
      }
      frame "DATABASE: SAVE DATABASE" {
        # "Your code here.\n(You can make a copy of, or modify, this frame)"
        n110 = Unbundle By Name(w314) -> ("Profile Creation"=w312:T1[], "Select Profile"=w306:path)
        n111 = Empty String/Path?(string/path=w306) -> (empty?=w307:bool)
        n112 = case shown="True" w307 {
          tunnel: w310 -> [w317 w326]
          tunnel: [w317 w325] -> w309
          tunnel: [w318 w319] -> w308
          tunnel: w306 -> [w318 _]
          frame False {
          }
          frame True {
            n113 = call "File Dialog"("error in"=w326) -> ("selected path"=w320:path, "error out"=w325:errorcluster)  [unwired: 11 in, 2 out]
            n114 = Strip Path(path=w320) -> (stripped path=w323:path, name=w322:string)
            n115 = Concatenate Strings(w322, ".txt") -> (w324:string)
            n116 = Build Path(base path=w323, name or relative path=w324) -> (appended path=w319:path)
          }
        }
        n117 = Write to Binary File(file (use dialog)=w308, data=w312, error in=w309) -> (error out=w311:errorcluster)  [unwired: 3 in, 2 out]
        n118 = flat-sequence {
          tunnel: [w328] -> w313
          tunnel: w311 -> [w328]
          frame #0 {
            n119 = One Button Dialog(message="Profile data is Saved") -> ()  [unwired: 1 in, 1 out]
          }
        }
        n120 = call <vilib>:"Add State(s) to Queue__JKI_lib_State_Machine.vi"("State(s) in (\"\")"=w316) -> ("States Out"=w315:string)  [unwired: 14 in]
      }
      frame "DATABASE: READ DATABASE" {
        # "Your code here.\n(You can make a copy of, or modify, this frame)"
        n121 = Unbundle By Name(w338) -> ("Profile Creation"=w333:T1[], "Select Profile"=w329:path)
        n122 = call <vilib>:"Check if File or Folder Exists.vi"("error in (no error)"=w336, "path"=w329) -> ("error out"=w334:errorcluster, "file or folder exists?"=w332:bool, "dup path"=w335:path)  [unwired: 7 in]
        n123 = case shown="True" w332 {
          tunnel: w335 -> [_ w349]
          tunnel: w334 -> [w342 w348]
          tunnel: [w342 w345] -> w331
          tunnel: w333 -> [_ w347]
          tunnel: [T1[] [] ("Profile Creation") w344] -> w330
          frame False {
            n124 = One Button Dialog(message="File Path not Found!") -> ()  [unwired: 1 in, 1 out]
          }
          frame True {
            n125 = Read from Binary File(5:w347, 8:w348, 11:w349) -> (0:w346:errorcluster, 2:w344:T1[])  [unwired: 3 in, 2 out]
            n126 = call <vilib>:"Simple Error Handler.vi"("error in (no error)"=w346) -> ("error out"=w345:errorcluster)  [unwired: 4 in, 4 out]
          }
        }
        n127 = Bundle By Name(cluster=w338, "Profile Creation"=w330) -> (w337:T4)
        n128 = call <vilib>:"Add State(s) to Queue__JKI_lib_State_Machine.vi"("State(s) in (\"\")"=w340) -> ("States Out"=w339:string)  [unwired: 14 in]
      }
    }
    n129 = Unbundle By Name(w13) -> ("Profile Creation"=w12:T1[])
    n130 = property on="Profile Creation" class="Arr (strict)"(error in=w15, "Value"=w12) -> (error out=w14:errorcluster)  [unwired: 1 in, 1 out]
  }
